vi "PH_Beamline.set Radiation Shutter Settings.vi"(0 "i ref in":refnum<vi>, 5 "error in":errorcluster) -> (14 "i ref out":refnum<vi>, 19 "error out":errorcluster)   [LabVIEW 2014, in "PH_Beamline.lvlib"]
uses:
  PH_Beamline.lvlib
  PH_Basics/PH_SystemInformation/PH_SystemInformationEnabling State.ctl
  PH_Basics/PH_SystemInformation/PH_SystemInformation.lvlib
  PH_BL-Master/PH_BL-Master.lvlib
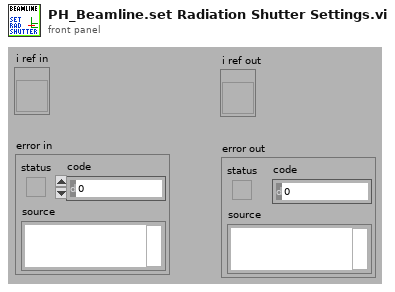
[diagram p1: front panel]
types:
  T1 = enum16{"Laser", "PreAmp", "MainAmp", "Exp 1", "Exp 2", "Exp 3", "Exp 4"}
  T2 = typedef "PH_SystemInformation.lvlib/PH_SystemInformationEnabling State.ctl" = i32
  T3 = typedef "PH_Beamline.lvlib/PH_Beamline.i attribute.ctl" = cluster{"GUI Refs":cluster{"PA ok":refnum<vi>, "MA ok":refnum<vi>, "fs FE ok":refnum<vi>, "ns FE ok":refnum<vi>, "PA ED ok":refnum<vi>, "MAS ok":refnum<vi>, "Booster ok":refnum<vi>, "Mirrortower ok":refnum<vi>, "In.-Box ok":refnum<vi>, "Compressor ok":refnum<vi>, "Experiment LB ok":refnum<vi>, "Experiment LL ok":refnum<vi>, "PHELIX_Beckhoff_Watchdog":refnum<vi>, "Shutters closed":refnum<vi>, "uOPA ok":refnum<vi>, "Vacuum no shotcond Comp LB":refnum<vi>}, "Refs BL MA":refnum<vi>[], "Refs BL MA-IB":refnum<vi>[], "Refs BL fs":refnum<vi>[], "Refs BL PA ED":refnum<vi>[], "Refs BL MAS":refnum<vi>[], "Refs BL Boo":refnum<vi>[], "Refs BL ns":refnum<vi>[], "Refs BL Mirrortower":refnum<vi>[], "Refs BL Compressor":refnum<vi>[], "Refs BL Exp LB":refnum<vi>[], "Radiation Safety":cluster{"Exp Laserbay":cluster{"Ref Op Mode":refnum<vi>, "Ref Laserbay evacuated":refnum<vi>, "Tagname LB evacuated":string, "Shot Mode":T4, "Laserbay evacuated?":i32, "Tagname HV room locked":string, "HV room locked?":i32, "Ref HV room locked":refnum<vi>, "Tagname bridged?":string, "Ref Bridge":refnum<vi>, "I<1E18W/cm²":bool}, "Exp Laserlab":cluster{"Ref Op Mode":refnum<vi>, "Ref Laserlab evacuated":refnum<vi>, "Tagname LL evacuated":string, "Shot Mode":T4, "Laserlab evacuated?":i32, "Tagname bridged?":string, "Ref Bridge":refnum<vi>, "I<1E18W/cm²":bool}}, "Refs BL LL":refnum<vi>[], "PP Igni Heating GUI Refs":refnum<vi>[], "PP Igni Heating Tagnames ":string[], "Refs BL PA":cluster{"undelayed Line before Shutter":refnum<vi>[], "undelayed Line after Shutter":refnum<vi>[], "before Bypass":refnum<vi>[], "delayed Line before Shutter":refnum<vi>[], "delayed Line after Shutter":refnum<vi>[], "before Shutter Input":refnum<vi>[], "after Shutter Input":refnum<vi>[], "Bypass":refnum<vi>[], "before Shutter Exit":refnum<vi>[], "after Shutter Exit":refnum<vi>[], "to MA":refnum<vi>[], "to Lab":refnum<vi>[]}, "BL":cluster{"YLF_BL_Status":i32, "fs_BL_Status":i32, "fs_YLF_BL_Status":i32, "ns_BL_Status":i32, "PA_Input_BL_Status":i32, "PA_UnDelay_BL_Status":i32, "PA_Delay_BL_Status":i32, "PA_BL_Status":i32, "PA_Bypass_BL_Status":i32, "PA_Exit_BL_Status":i32, "PA_LL_BL_Status":i32, "LL_BL_Status":i32, "PA_MA_BL_Status":i32, "MA_Exit_BL_Status":i32, "MA_Z6_BL_Status":i32, "Z6_BL_Status":i32, "MA_LB_BL_Status":i32, "LB_TB2_BL_Status":i32, "PA_before_Bypass_BL_Status":i32, "LB_TB3_BL_Status":i32}, "State Subsystems":cluster{"PA":bool, "MA":bool, "ns FE":bool, "fs FE":bool, "PA ED":bool, "In.-Box":bool, "MAS":bool, "Booster":bool, "Mirrortower":bool, "Compressor":bool, "Experiment LB":bool, "Experiment LL":bool, "uOPA":bool}, "Status Subscriber Information":T5, "Refs BL uOPA":refnum<vi>[], "PA_Input_2_Beam_6PWpGUI not linked?":bool, "PA_Input_Delay_6PGUI not linked?":bool, "Settings":T8}
  T4 = typedef "PH_Beamline.lvlib/PH_Beamline.Operation Mode.ctl" = i32
  T5 = typedef "PH_Beamline.lvlib/PH_Beamline.Status Subscriber Information.ctl" = cluster{"fs Swich YLF":T6, "fs Exit Shutter":T6, "ns Exit Shutter":T6, "PA Input Shutter":T6, "PA PC WP":T6, "PA PC WP 2":T6, "PA Bypass In":T6, "PA Bypass Out":T6, "PA CH 1":T6, "PA delayed":T6, "PA non delayed":T6, "PA Exit Shutter":T6, "PA Switch Lab":T6, "PA Bridge CH Input MA":T6, "MA Diffusor IB":T6, "MA IB Ready":T6, "MA CH 1":T6, "MA CH 2":T6, "MA CH 3":T6, "MA CH 4":T6, "MA Shutter Align Cam":T6, "MA Position MM5":T6, "Calorimeter Switch":T6, "BL Z6 CH 9":T6, "BL Z6 Beamdump":T6, "BL Z6 Shutter":T6, "COS Sensitivity Switch":T6, "Exp LB Shutter":T6, "Exp LB TB 2":T6, "Exp LB TB 3":T6, "PA LL Input CH":T6, "PA LL Output CH":T6, "LL Comp Input Shutter":T6, "LL Comp Output Shutter":T6, "LL Comp FF Shutter":T6, "Exp LL Shutter":T6, "MA IM In IB":T6, "MA IM Out IB":T6, "MA DB In IB":T6, "MA DB Out IB":T6, "Exp LB Shutter Interlock":T6, "Exp LL Shutter Interlock":T6, "MM1 Force Sensor":T6}
  T6 = typedef "PH_BL-Master.lvlib/PH_BL-Master.Status Subscriber Information.ctl" = cluster{"Index of element":i32, "Attributeset":T7}
  T7 = typedef "PH_BL-Master.lvlib/PH_BL-Master.Attribute Set.ctl" = enum16{"Boolean Status Service Subscriber", "Picture Status Service Subscriber"}
  T8 = typedef "PH_Beamline_Chief.lvlib/PH_Beamline_Chief.Settings.ctl" = cluster{"PA Doublepass Mode":bool, "Compressor Vaccuum LB not relevant":bool, "Windowshutter TB2 not relevant":bool, "Windowshutter TB3 not relevant":bool}
  T9 = enum8{"Enabled", "Disabled", "Disabled and Grayed Out"}
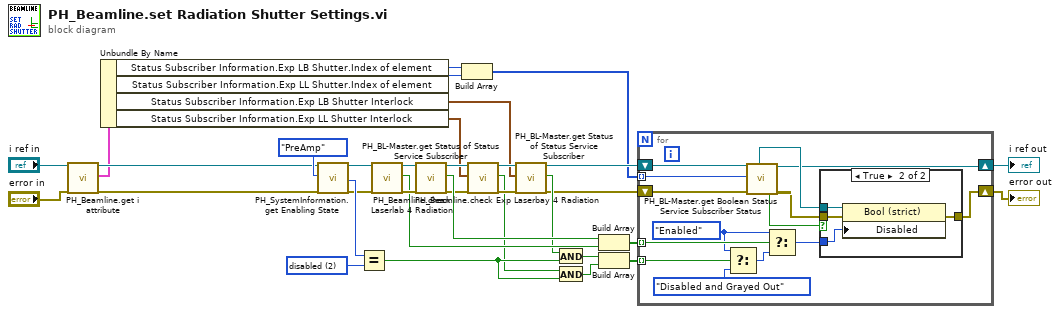
[diagram p0: block diagram]
diagram:
  w32 = T2 2 items=["no info", "not disabled", "disabled"] ("PreAmp Enabling State")
  n1 = call "PH_Beamline.get i attribute.vi"("i ref in"="i ref in", "error in (no error)"="error in") -> ("i ref out"=w9:refnum<vi>, "i attribute"=w6:T3, "error out"=w7:errorcluster)  [unwired: 15 in]
  n2 = Unbundle By Name(w6) -> ("Status Subscriber Information.Exp LB Shutter.Index of element"=w5:i32, "Status Subscriber Information.Exp LL Shutter.Index of element"=w4:i32, "Status Subscriber Information.Exp LB Shutter Interlock"=w2:T6, "Status Subscriber Information.Exp LL Shutter Interlock"=w1:T6)
  n3 = call "PH_SystemInformation.get Enabling State.vi"("i ref in"=w9, "Wanted State"=T1."PreAmp", "error in (no error)"=w7) -> ("i ref out"=w30:refnum<vi>, "Enabling State"=w33:T2, "error out"=w28:errorcluster)  [unwired: 14 in]
  n4 = Equal?(x=w33, y=w32) -> (x = y?=w16:bool)
  n5 = call "PH_Beamline.check Laserlab 4 Radiation.vi"("i ref in"=w30, "error in"=w28) -> ("i ref out"=w29:refnum<vi>, "Laserlab save concerning Radiation"=w26:bool, "error out"=w27:errorcluster)  [unwired: 15 in]
  n6 = call "PH_Beamline.check Exp Laserbay 4 Radiation.vi"("i ref in"=w29, "error in"=w27) -> ("i ref out"=w20:refnum<vi>, "Laserbay save concerning Radiation"=w25:bool, "error out"=w18:errorcluster)  [unwired: 15 in]
  n7 = Build Array(w5, w4) -> (w3:i32[])
  n8 = call "PH_BL-Master.get Status of Status Service Subscriber.vi"("i ref in"=w20, "Wanted Status Subscriber Information"=w1, "error in (no error)"=w18) -> ("i ref out"=w19:refnum<vi>, "on/true/in?"=w14:bool, "error out"=w17:errorcluster)  [unwired: 11 in, 3 out]
  n9 = call "PH_BL-Master.get Status of Status Service Subscriber.vi"("i ref in"=w19, "Wanted Status Subscriber Information"=w2, "error in (no error)"=w17) -> ("i ref out"=w11:refnum<vi>, "on/true/in?"=w23:bool, "error out"=w12:errorcluster)  [unwired: 11 in, 3 out]
  n10 = And(x=w23, y=w16) -> (x .and. y?=w22:bool)
  n11 = And(x=w14, y=w16) -> (x .and. y?=w15:bool)
  n12 = Build Array(w25, w26) -> (w24:bool[])
  n13 = Build Array(w22, w15) -> (w21:bool[])
  n14 = for {
    shift-right: [w48] -> w31
    shift-left: w12 -> [w41]
    tunnel: w3 -> [w40] mode=indexing
    tunnel: w21 -> [w46] mode=indexing
    tunnel: w24 -> [w45] mode=indexing
    shift-right: [w35] -> w10
    shift-left: w11 -> [w36]
    w42 = T9."Enabled" ("Disabled")
    n15 = Select(t=w42, s=w46, f=T9."Disabled and Grayed Out" ("Disabled")) -> (s? t:f=w47:T9)
    n16 = call "PH_BL-Master.get Boolean Status Service Subscriber Status.vi"("i ref in"=w36, "Index of wanted element"=w40, "error in (no error)"=w41) -> ("Wanted Boolean Ref"=w39:refnum<vi>, "Information found?"=w37:bool, "i ref out"=w35:refnum<vi>, "error out"=w38:errorcluster)  [unwired: 8 in, 5 out]
    n17 = Select(t=w42, s=w45, f=w47) -> (s? t:f=w44:T9)
    n18 = case shown="True" w37 {
      tunnel: [w49 w53] -> w48
      tunnel: w38 -> [w49 w52]
      tunnel: w39 -> [_ w51]
      tunnel: w44 -> [_ w50]
      frame False {
      }
      frame True {
        n19 = property class="Bool (strict)"(reference=w51, error in=w52, "Disabled"=w50) -> (error out=w53:errorcluster)  [unwired: 1 out]
      }
    }
  }
  "error out" <- w31
  "i ref out" <- w10
